vi "Monitor_Cliente_Consumidor_v2.vi"() -> ()   [LabVIEW 2024]
uses:
  controls/Menu_States.ctl
panel:
  out "Heater Lebel [V]":dbl
  out "Temp. Display":T1(graph)
  out "Boolean":bool
  out "Enum":T2=enum."Measure"
  in  "User Control":T3
  out "Temp [ºC]":dbl(slide) scale=0.0..100.0
  out "Estado":string="int"
  out "Ventilator":bool
  out "Historic Data":T4
  out "HEATER":string
  in  "Start Acq":bool=TRUE
  in  "Quit":bool
  in  "Stop Acq":bool
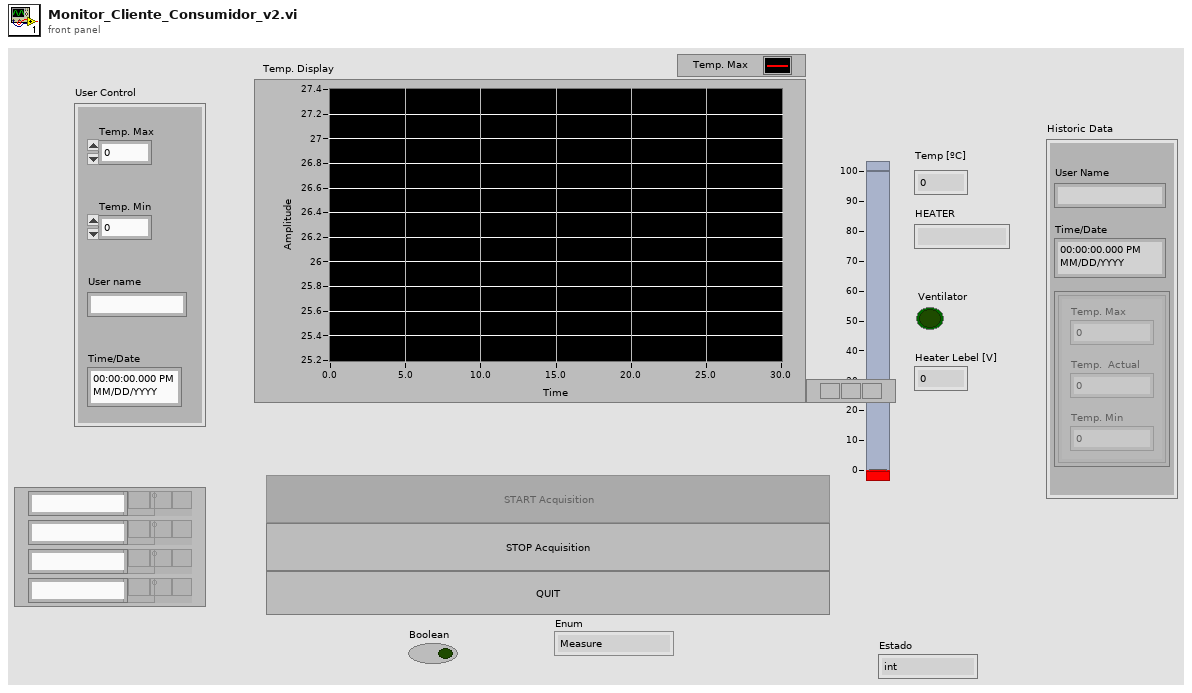
[diagram p1: front panel]
types:
  T1 = cluster{"Temp. Max":dbl, "Temp. Min":dbl, "RTD Temp":dbl}
  T2 = typedef "Menu_States.ctl" = enum8{"Initialize", "Measure", "Cooling", "Maximum", "Medium", "View Acquired Data", "Quit"}
  T3 = cluster{"Temp. Max":dbl, "Temp. Min":dbl, "User name":string, "Time/Date":timestamp}
  T4 = cluster{"User Name":string, "Time/Date":timestamp, "Array":cluster{"Temp. Max":dbl, "Temp.  Actual":dbl, "Temp. Min":dbl}[]}
  T5 = enum8{"Enabled", "Disabled", "Disabled and Grayed Out"}
  T6 = cluster{"RTD Temp":dbl, "Temp. Max":dbl, "Temp. Min":dbl}
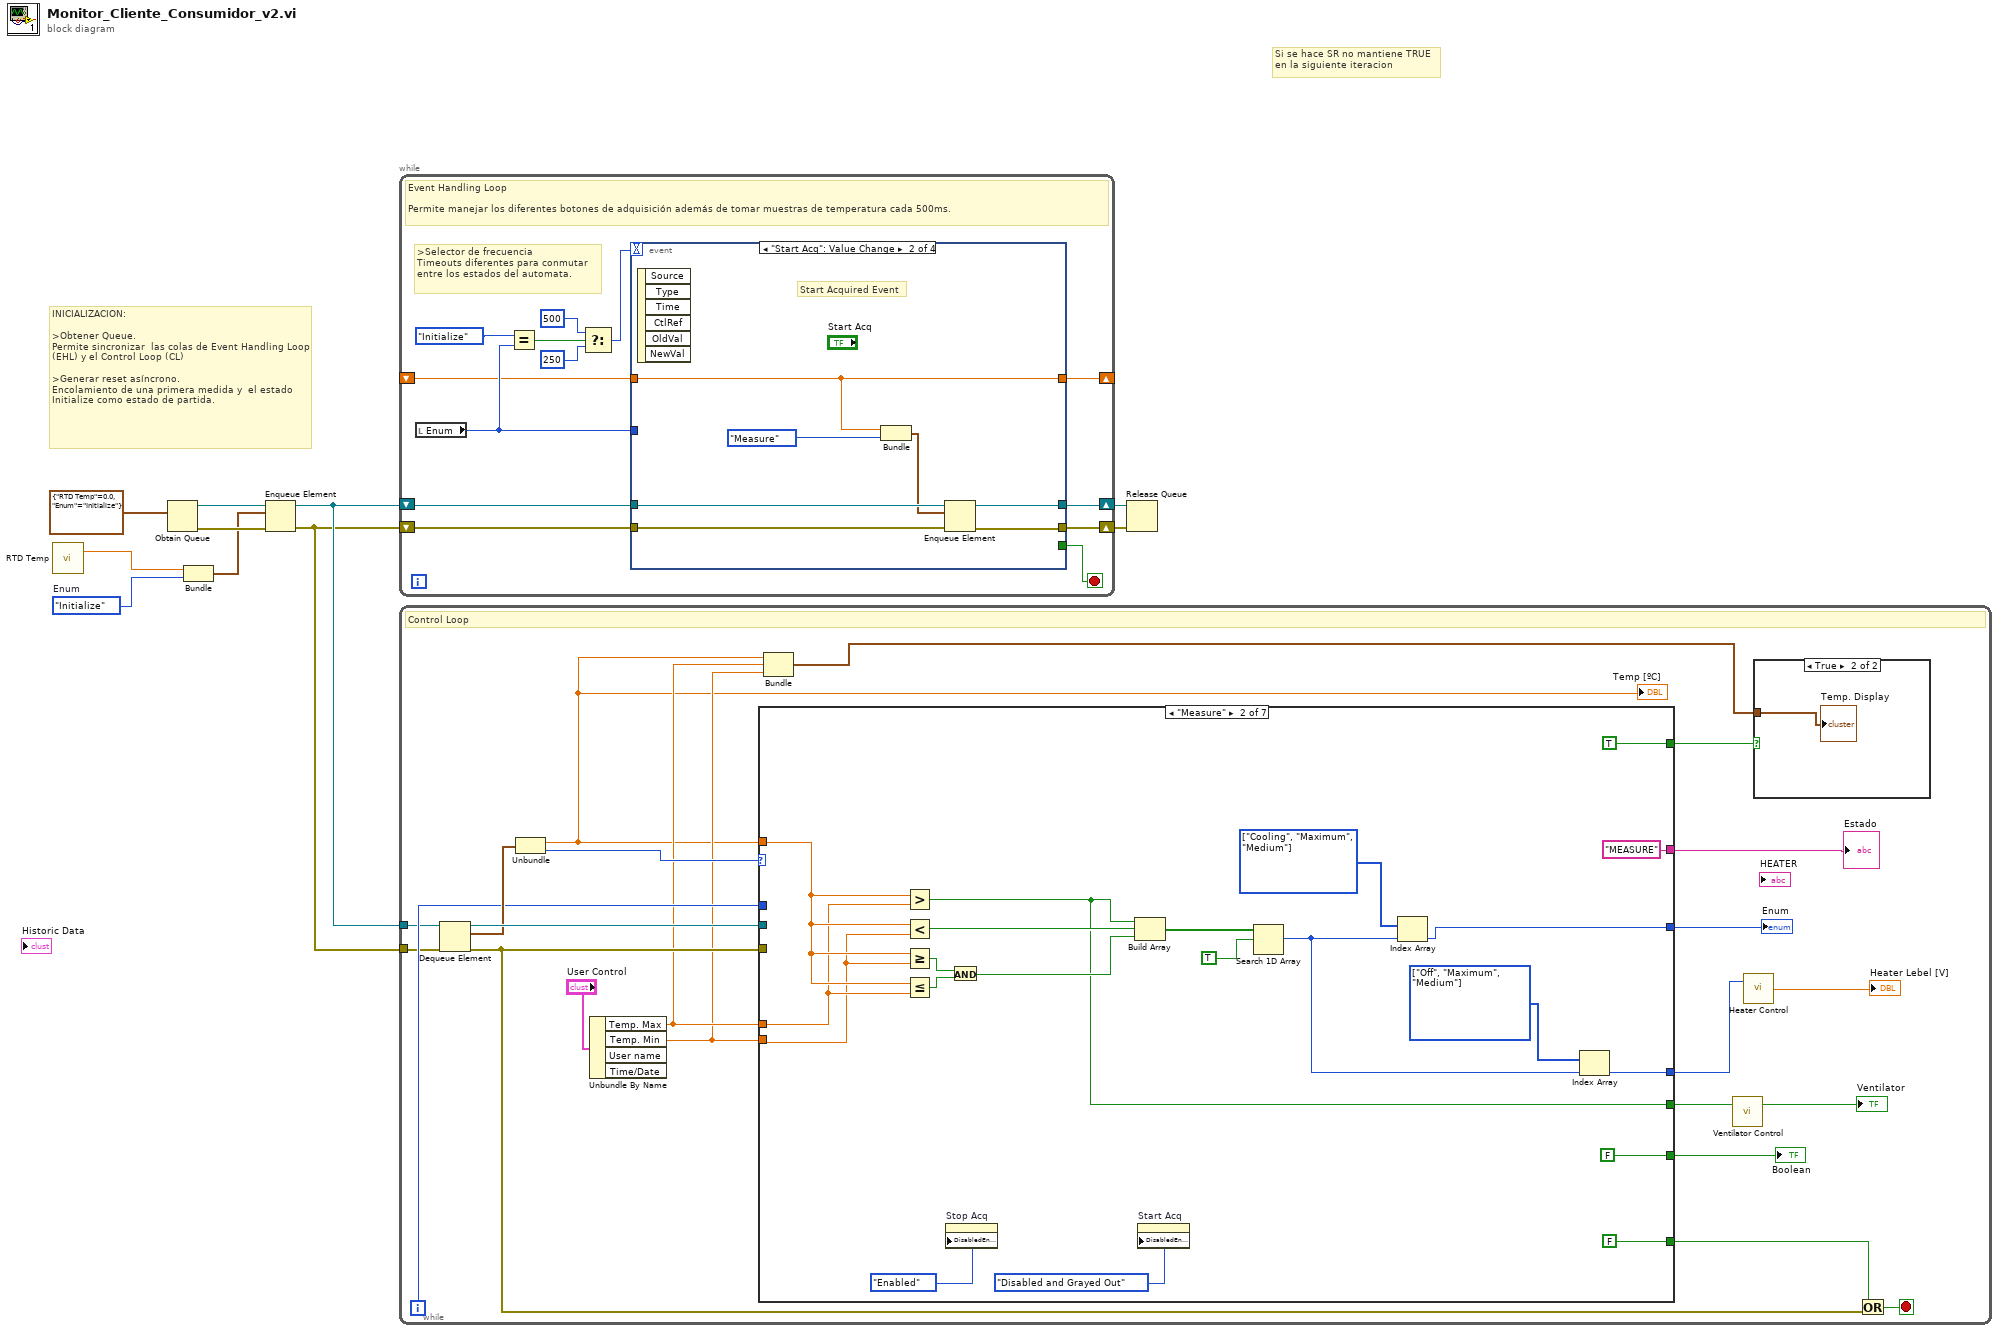
[diagram p0: block diagram]
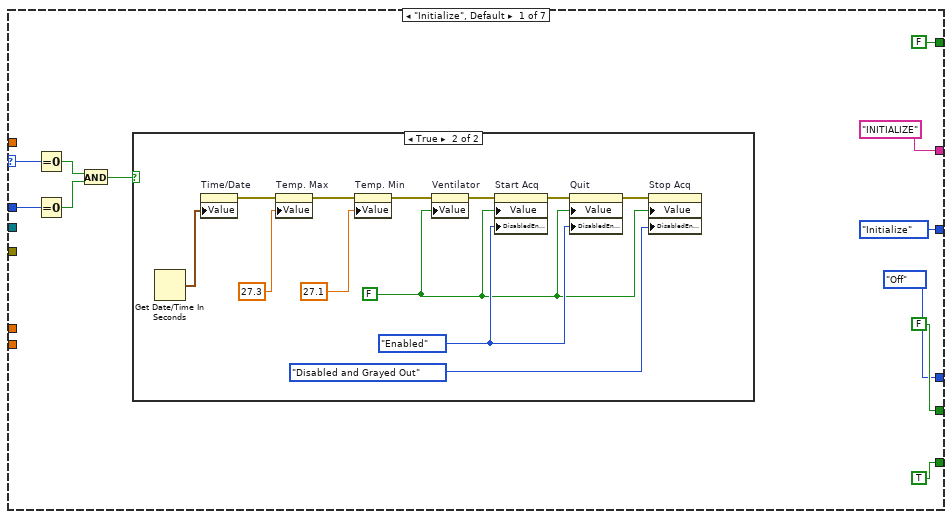
[diagram p3: hidden frame]
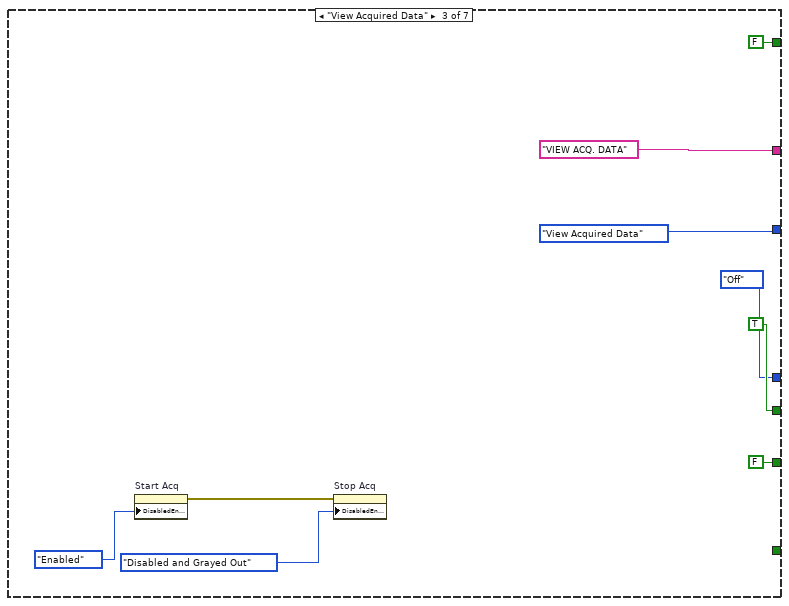
[diagram p5: hidden frame]
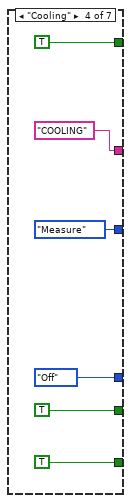
[diagram p6: hidden frame]
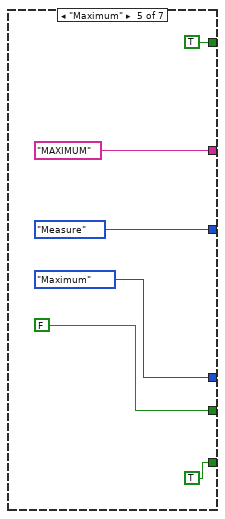
[diagram p7: hidden frame]
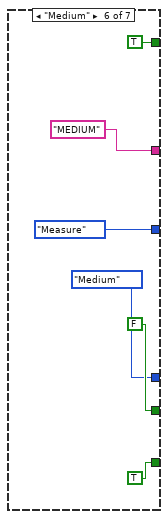
[diagram p8: hidden frame]
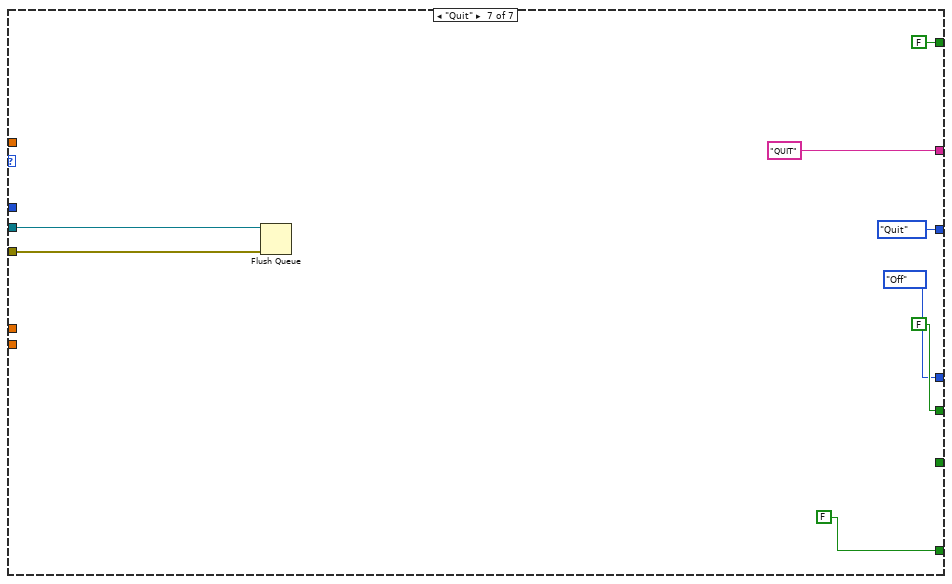
[diagram p9: hidden frame]
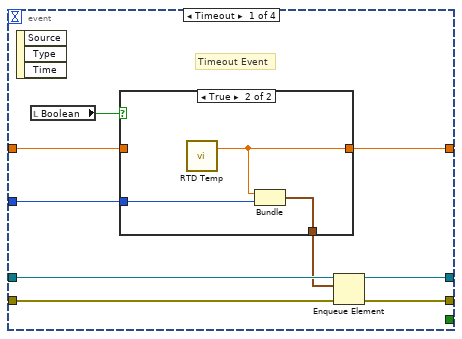
[diagram p10: hidden frame]
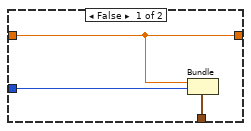
[diagram p11: hidden frame]
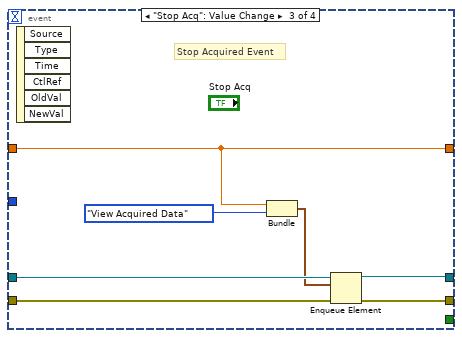
[diagram p12: hidden frame]
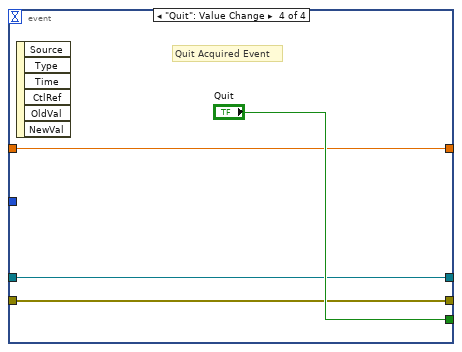
[diagram p13: hidden frame]
diagram:
  w1 = Menu_States."Initialize"  # Enum
  # "INICIALIZACION:\n\n>Obtener Queue.\nPermite sincronizar  las colas de Event Handling Loop (EHL) y el Control Loop (CL)\n\n>Generar reset asíncrono.\nEncolamiento de una primera medida y  el estado Initialize como estado de partida."
  # "Si se hace SR no mantiene TRUE\nen la siguiente iteracion"
  n1 = call "RTD Temp.vi"() -> ("RTD Temp"=w2:dbl)  [unwired: 1 in, 1 out]
  n2 = Obtain Queue(element data type=cluster{"RTD Temp":dbl, "Enum":T2} {"RTD Temp"=0.0, "Enum"=enum."Initialize"} ("output cluster")) -> (queue out=w8:refnum<queue>, error out=w6:errorcluster)  [unwired: 4 in, 1 out]
  n3 = Bundle("RTD Temp"=w2, "Enum"=w1) -> (w5:cluster{"RTD Temp":dbl, "Enum":T2})  [unwired: 1 in]
  n4 = Enqueue Element(queue=w8, element=w5, error in (no error)=w6) -> (queue out=w7:refnum<queue>, error out=w3:errorcluster)  [unwired: 1 in, 1 out]
  n5 = while {
    shift-right: [w20] -> w10
    shift-left: w7 -> [w23]
    shift-right: [w21] -> w9
    shift-left: w3 -> [w22]
    shift-right: [w12] -> _
    shift-left: _ -> [w11]
    stop <- w19 stop-if-true
    # ">Selector de frecuencia\nTimeouts diferentes para conmutar entre los estados del automata."
    # "Event Handling Loop\n\nPermite manejar los diferentes botones de adquisición además de tomar muestras de temperatura cada 500ms."
    n6 = local read "Enum"() -> (w18:T2)
    n7 = Equal?(x=Menu_States."Initialize" ("Enum"), y=w18) -> (x = y?=w14:bool)
    n8 = Select(t=500, s=w14, f=250) -> (s? t:f=w16:i32)
    n9 = event shown="[1] \"Start Acq\": Value Change" {
      selector: _ -> [_ _ _ _]
      dyn-events: _ -> [_ _ _ _]
      timeout: w16 -> [_ _ _ _]
      tunnel: w23 -> [w32 w45 w51 w54]
      tunnel: w22 -> [w31 w43 w49 w53]
      tunnel: [w29 w42 w48 w53] -> w21
      tunnel: [w30 w44 w50 w54] -> w20
      tunnel: [_ _ _ "Quit"] -> w19
      tunnel: w18 -> [w27 _ _ _]
      tunnel: [w25 w39 w46 w55] -> w12
      tunnel: w11 -> [w24 w39 w46 w55]
      event Timeout {
        # "Timeout Event"
        n10 = event-data() -> ()  [unwired: 1 in, 3 out]
        n11 = local read "Boolean"() -> (w26:bool)
        n12 = case shown="True" w26 {
          tunnel: [w34 w38] -> w28
          tunnel: w27 -> [w35 w37]
          tunnel: [w33 w36] -> w25
          tunnel: w24 -> [w33 _]
          frame False {
            n13 = Bundle("RTD Temp"=w33, "Enum"=w35) -> (w34:cluster{"RTD Temp":dbl, "Enum":T2})  [unwired: 1 in]
          }
          frame True {
            n14 = call "RTD Temp.vi"() -> ("RTD Temp"=w36:dbl)  [unwired: 1 in, 1 out]
            n15 = Bundle("RTD Temp"=w36, "Enum"=w37) -> (w38:cluster{"RTD Temp":dbl, "Enum":T2})  [unwired: 1 in]
          }
        }
        n16 = Enqueue Element(queue=w32, element=w28, error in (no error)=w31) -> (queue out=w30:refnum<queue>, error out=w29:errorcluster)  [unwired: 1 in, 1 out]
      }
      event "Start Acq": Value Change {
        # "Start Acquired Event"
        n17 = event-data() -> ()  [unwired: 1 in, 6 out]
        n18 = Bundle("RTD Temp"=w39, "Enum"=Menu_States."Measure") -> (w41:cluster{"RTD Temp":dbl, "Enum":T2})  [unwired: 1 in]
        n19 = Enqueue Element(queue=w45, element=w41, error in (no error)=w43) -> (queue out=w44:refnum<queue>, error out=w42:errorcluster)  [unwired: 1 in, 1 out]
      }
      event "Stop Acq": Value Change {
        # "Stop Acquired Event"
        n20 = event-data() -> ()  [unwired: 1 in, 6 out]
        n21 = Bundle("RTD Temp"=w46, "Enum"=Menu_States."View Acquired Data") -> (w47:cluster{"RTD Temp":dbl, "Enum":T2})  [unwired: 1 in]
        n22 = Enqueue Element(queue=w51, element=w47, error in (no error)=w49) -> (queue out=w50:refnum<queue>, error out=w48:errorcluster)  [unwired: 1 in, 1 out]
      }
      event "Quit": Value Change {
        # "Quit Acquired Event"
        n23 = event-data() -> ()  [unwired: 1 in, 6 out]
      }
    }
  }
  n24 = while {
    tunnel: w7 -> [w58]
    tunnel: w3 -> [w57]
    i -> [w71]
    stop <- w78 stop-if-true
    # "Control Loop"
    n25 = Dequeue Element(queue=w58, error in (no error)=w57) -> (queue out=w76:refnum<queue>, element=w73:cluster{"RTD Temp":dbl, "Enum":T2}, error out=w74:errorcluster)  [unwired: 1 in, 1 out]
    n26 = Unbundle(w73) -> ("RTD Temp"=w63:dbl, "Enum"=w70:T2)
    "Temp [ºC]" <- w63
    n27 = Unbundle By Name("User Control") -> ("Temp. Max"=w65:dbl, "Temp. Min"=w64:dbl)  [unwired: 2 out]
    n28 = case shown="\"Measure\"" w70 {
      selector: w70 -> [w89 _ _ _ _ _ _]
      tunnel: [_ FALSE _ _ _ _ FALSE] -> w77
      tunnel: w76 -> [_ _ _ _ _ _ w157]
      tunnel: w74 -> [_ _ _ _ _ _ w156]
      tunnel: ["INITIALIZE" "MEASURE" "VIEW ACQ. DATA" "COOLING" "MAXIMUM" "MEDIUM" "QUIT"] -> w75
      tunnel: w63 -> [_ w111 _ _ _ _ _]
      tunnel: w65 -> [_ w110 _ _ _ _ _]
      tunnel: w64 -> [_ w109 _ _ _ _ _]
      tunnel: w71 -> [w88 _ _ _ _ _ _]
      tunnel: [Menu_States."Initialize" ("Enum") w112 Menu_States."View Acquired Data" ("Enum") Menu_States."Measure" ("Enum") Menu_States."Measure" ("Enum") Menu_States."Measure" ("Enum") Menu_States."Quit" ("Enum")] -> w69
      tunnel: [TRUE ("Boolean") FALSE ("Boolean") FALSE ("Boolean") TRUE ("Boolean") TRUE ("Boolean") TRUE ("Boolean") _] -> w68
      tunnel: [FALSE ("Ventilator (off)") w106 TRUE ("Ventilator (off)") TRUE ("Ventilator (off)") FALSE ("Ventilator (off)") FALSE ("Ventilator (off)") FALSE ("Ventilator (off)")] -> w66
      tunnel: [enum16{"Off", "Medium", "Maximum"}."Off" ("Heater Level") w104 enum16{"Off", "Medium", "Maximum"}."Off" ("Heater Level") enum16{"Off", "Medium", "Maximum"}."Off" ("Heater Level") enum16{"Off", "Medium", "Maximum"}."Maximum" ("Heater Level") enum16{"Off", "Medium", "Maximum"}."Medium" ("Heater Level") enum16{"Off", "Medium", "Maximum"}."Off" ("Heater Level")] -> w62
      tunnel: [FALSE TRUE FALSE TRUE TRUE TRUE FALSE] -> w59
      frame "Initialize", Default {
        n29 = Equal To 0?(x=w89) -> (x = 0?=w87:bool)
        n30 = Equal To 0?(x=w88) -> (x = 0?=w86:bool)
        n31 = And(x=w87, y=w86) -> (x .and. y?=w85:bool)
        n32 = case shown="True" w85 {
          frame False {
          }
          frame True {
            w93 = T5."Enabled" ("Disabled")
            w91 = FALSE ("Ventilator")
            n33 = Get Date/Time In Seconds() -> (seconds since 1Jan1904=w102:timestamp)
            n34 = property on="Time/Date" class="AbsTime (strict)"("Value"=w102) -> (error out=w99:errorcluster)  [unwired: 2 in, 1 out]
            n35 = property on="Temp. Max" class="DigNum (strict)"(error in=w99, "Value"=27.3) -> (error out=w98:errorcluster)  [unwired: 1 in, 1 out]
            n36 = property on="Temp. Min" class="DigNum (strict)"(error in=w98, "Value"=27.1) -> (error out=w97:errorcluster)  [unwired: 1 in, 1 out]
            n37 = property on="Ventilator" class="Bool (strict)"(error in=w97, "Value"=w91) -> (error out=w96:errorcluster)  [unwired: 1 in, 1 out]
            n38 = property on="Start Acq" class="Bool (strict)"(error in=w96, "Value"=w91, "DisabledEnum"=w93) -> (error out=w95:errorcluster)  [unwired: 1 in, 1 out]
            n39 = property on="Quit" class="Bool (strict)"(error in=w95, "Value"=w91, "DisabledEnum"=w93) -> (error out=w94:errorcluster)  [unwired: 1 in, 1 out]
            n40 = property on="Stop Acq" class="Bool (strict)"(error in=w94, "Value"=w91, "DisabledEnum"=T5."Disabled and Grayed Out" ("Disabled")) -> ()  [unwired: 1 in, 2 out]
          }
        }
      }
      frame "Measure" {
        w105 = enum16{"Off", "Medium", "Maximum"}[] [enum."Off", enum."Maximum", enum."Medium"] items=["Off", "Medium", "Maximum"] ("Heater Level")
        w113 = T2[] [enum."Cooling", enum."Maximum", enum."Medium"] items=["Initialize", "Measure", "Cooling", "Maximum", "Medium", "View Acquired Data", "Quit"] ("array")
        n41 = Greater?(x=w111, y=w110) -> (0:w106:bool)
        n42 = Less?(x=w111, y=w109) -> (x < y?=w117:bool)
        n43 = Greater Or Equal?(x=w111, y=w109) -> (x >= y?=w116:bool)
        n44 = Less Or Equal?(x=w111, y=w110) -> (x <= y?=w115:bool)
        n45 = property on="Stop Acq" class="Bool (strict)"("DisabledEnum"=T5."Enabled" ("Disabled")) -> ()  [unwired: 2 in, 2 out]
        n46 = And(x=w116, y=w115) -> (x .and. y?=w114:bool)
        n47 = Build Array(w106, w117, w114) -> (w119:bool[])
        n48 = property on="Start Acq" class="Bool (strict)"("DisabledEnum"=T5."Disabled and Grayed Out" ("Disabled")) -> ()  [unwired: 2 in, 2 out]
        n49 = Search 1D Array(1D array=w119, element=TRUE) -> (index of element=w103:i32)  [unwired: 1 in]
        n50 = Index Array(array=w113, index=w103) -> (element=w112:T2)
        n51 = Index Array(array=w105, index=w103) -> (element=w104:enum16{"Off", "Medium", "Maximum"})
      }
      frame "View Acquired Data" {
        n52 = property on="Start Acq" class="Bool (strict)"("DisabledEnum"=T5."Enabled" ("Disabled")) -> (error out=w130:errorcluster)  [unwired: 2 in, 1 out]
        n53 = property on="Stop Acq" class="Bool (strict)"(error in=w130, "DisabledEnum"=T5."Disabled and Grayed Out" ("Disabled")) -> ()  [unwired: 1 in, 2 out]
      }
      frame "Cooling" {
      }
      frame "Maximum" {
      }
      frame "Medium" {
      }
      frame "Quit" {
        n54 = Flush Queue(queue=w157, error in (no error)=w156) -> ()  [unwired: 3 out]
      }
    }
    "Estado" <- w75
    "Enum" <- w69
    "Boolean" <- w68
    n55 = Bundle("RTD Temp"=w63, "Temp. Max"=w65, "Temp. Min"=w64) -> (w60:T6)  [unwired: 1 in]
    n56 = call "Ventilator Control.vi"("Ventilator (off)"=w66) -> ("Ventilator State"=→"Ventilator":bool)  [unwired: 1 in, 1 out]
    n57 = call "Heater Control.vi"("Heater Level"=w62) -> ("Heater Level (V)"=→"Heater Lebel [V]":dbl)  [unwired: 2 in, 1 out]
    n58 = case shown="True" w59 {
      tunnel: w60 -> [_ w79]
      frame False {
      }
      frame True {
        "Temp. Display" <- w79
      }
    }
    n59 = Or(x=w77, y=w74) -> (x .or. y?=w78:bool)
  }
  n60 = Release Queue(queue=w10, error in (no error)=w9) -> ()  [unwired: 1 in, 3 out]
